vi "IZMoveDown.vi"(0 "PRIORLib.IZIn":refnum<k7>, 1 "Distance":dbl=100.0) -> (2 "PRIORLib.IZOut":refnum<k7>, 3 "error out":errorcluster, 4 "Return":i32)   [LabVIEW 2011]
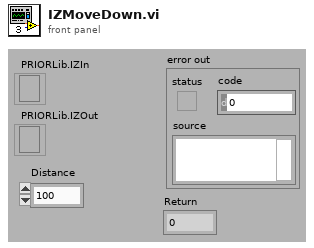
[diagram p1: front panel]
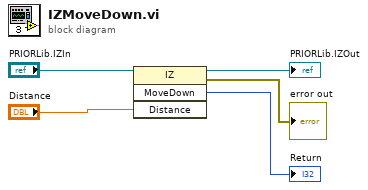
[diagram p0: block diagram]
diagram:
  n1 = invoke class="IZ" method="MoveDown"(reference="PRIORLib.IZIn", "Distance"="Distance") -> (reference out=→"PRIORLib.IZOut":refnum<k7>, error out=→"error out":errorcluster, "MoveDown"=→"Return":i32)  [unwired: 2 in, 1 out]
